vi "CRYProject Editor PIC Signal Project Function.vi"(10 "sData":string="Save As") -> ()   [LabVIEW 2013]
uses:
  CRYProject Editor Global.vi
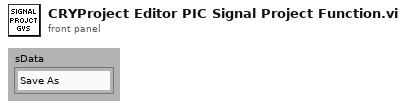
[diagram p1: front panel]
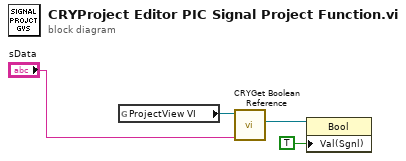
[diagram p0: block diagram]
diagram:
  n1 = global read "CRYProject Editor Global.vi" "ProjectView VI"() -> (w4:refnum<vi>)
  n2 = call "CRYGet Boolean Reference.vi"("Label Name"="sData", "VI Refnum"=w4) -> ("Boolean Ref"=w3:refnum<vi>)  [unwired: 7 in, 2 out]
  n3 = property class="Bool"(reference=w3, "Val(Sgnl)"=TRUE) -> ()  [unwired: 1 in, 2 out]
